vi "舵机(子VI1).vi"(9 "车速控制":dbl(slide) scale=-1.0..1.0, 10 "舵机":dbl(slide) min=-100.0 max=100.0 scale=-200.0..200.0, 11 "null offset输入":bool) -> ()   [LabVIEW 2014]
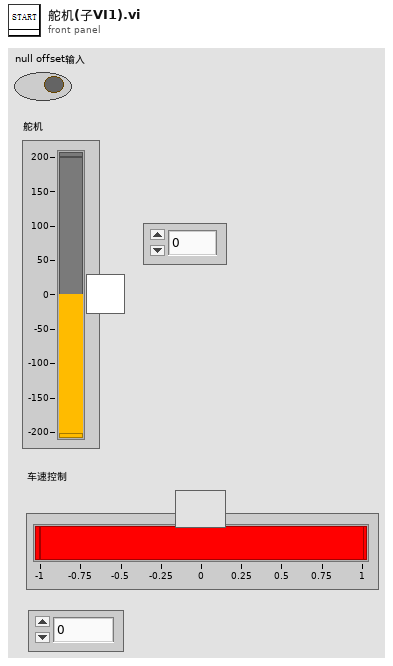
[diagram p1: front panel]
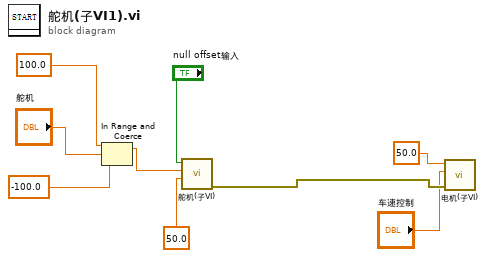
[diagram p0: block diagram]
diagram:
  n1 = In Range and Coerce(upper limit=100.0 ("上限"), x="舵机", lower limit=-100.0 ("下限")) -> (coerced(x)=w7:dbl)  [unwired: 1 out]
  n2 = call "舵机(子VI).vi"("freq [Hz]"=50.0, "舵机"=w7, "null offset"="null offset输入") -> ("error out"=w5:errorcluster)  [unwired: 5 in, 3 out]
  n3 = call "电机(子VI).vi"("error in (no error)"=w5, "车速控制"="车速控制", "hz"=50.0) -> ()  [unwired: 8 in, 1 out]
